vi "MakeCall.vi"(8 "error in (no error)":errorcluster, 11 "Customer With Cell Phone in":refnum<class "Customer With Cell Phone.lvclass">) -> (0 "error out":errorcluster, 3 "Customer With Cell Phone out":refnum<class "Customer With Cell Phone.lvclass">)   [LabVIEW 2023, in "Customer With Cell Phone.lvlib" / "Customer With Cell Phone.lvclass"]
doc: "Simulates a phone call. A customer on a phone call will not respond to any other message until the phone call is complete."
uses:
  Customer With Cell Phone.lvclass
panel:
  in  "On cell phone":string="On cell phone"
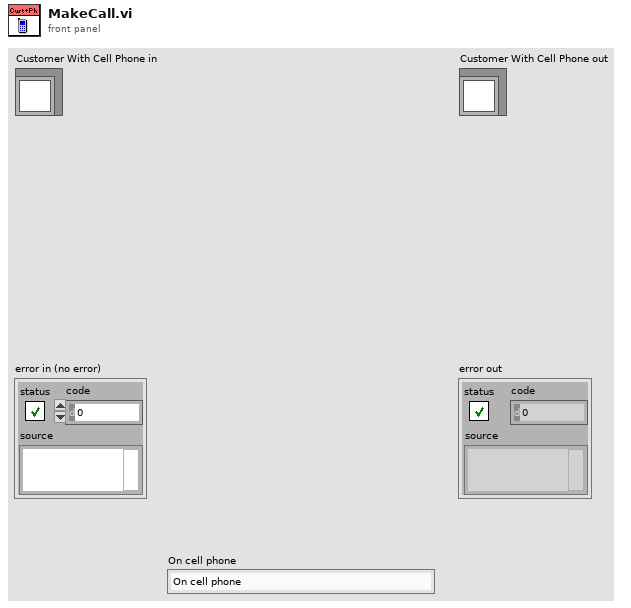
[diagram p1: front panel]
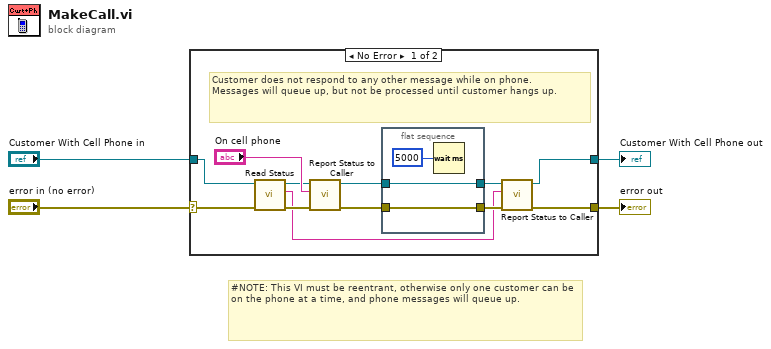
[diagram p0: block diagram]
diagram:
  # "#NOTE: This VI must be reentrant, otherwise only one customer can be on the phone at a time, and phone messages will queue up."
  n1 = case shown="No Error" "error in (no error)" {
    selector: "error in (no error)" -> [w9 w21]
    tunnel: [w10 w21] -> w3
    tunnel: [w11 w20] -> w1
    tunnel: "Customer With Cell Phone in" -> [w6 w20]
    frame No Error {
      # "Customer does not respond to any other message while on phone.\nMessages will queue up, but not be processed until customer hangs up."
      n2 = call-dynamic "Read Status.vi"("error in (no error)"=w9, "Customer in"=w6) -> ("error out"=w8:errorcluster, "Status"=w5:string, "Customer out"=w7:refnum<class "Customer With Cell Phone.lvclass">)  [unwired: 7 in]
      n3 = call-dynamic "Report Status to Caller.vi"("error in"=w8, "Status"="On cell phone", "Customer in"=w7) -> ("error out"=w14:errorcluster, "Customer out"=w15:refnum<class "Customer With Cell Phone.lvclass">)  [unwired: 7 in]
      n4 = flat-sequence {
        tunnel: w15 -> [w18]
        tunnel: [w18] -> w12
        tunnel: w14 -> [w17]
        tunnel: [w17] -> w13
        frame #0 {
          n5 = Wait (ms)(milliseconds to wait=u32 5000) -> ()  [unwired: 1 out]
        }
      }
      n6 = call-dynamic "Report Status to Caller.vi"("error in"=w13, "Status"=w5, "Customer in"=w12) -> ("error out"=w10:errorcluster, "Customer out"=w11:refnum<class "Customer With Cell Phone.lvclass">)  [unwired: 7 in]
    }
    frame Error {
    }
  }
  "error out" <- w3
  "Customer With Cell Phone out" <- w1
